vi "Read Pin Map File Contents.vi"(8 "error in":errorcluster, 11 "pin map file path":path) -> (0 "error out":errorcluster, 3 "pin map xml":string)   [LabVIEW 2021, in "NI Pin Map V1 Client.lvlib"]
uses:
  NI Pin Map V1 Client.lvlib
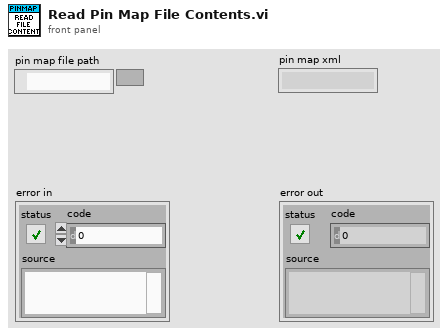
[diagram p1: front panel]
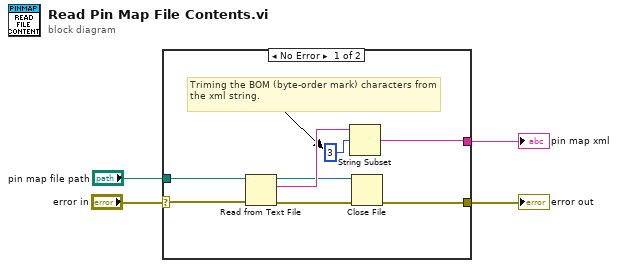
[diagram p0: block diagram]
diagram:
  n1 = case shown="No Error" "error in" {
    selector: "error in" -> [w12 w13]
    tunnel: "pin map file path" -> [w11 _]
    tunnel: [w5 w13] -> w1
    tunnel: [w8 _] -> w2
    frame No Error {
      # "Triming the BOM (byte-order mark) characters from the xml string."
      n2 = Read from Text File(file (use dialog)=w11, error in=w12) -> (refnum out=w7:refnum<file>, text=w10:string, error out=w6:errorcluster)  [unwired: 2 in, 1 out]
      n3 = String Subset(string=w10, offset (0)=3) -> (substring=w8:string)  [unwired: 1 in]
      n4 = Close File(refnum=w7, error in=w6) -> (error out=w5:errorcluster)  [unwired: 1 out]
    }
    frame Error {
    }
  }
  "pin map xml" <- w2
  "error out" <- w1
